vi "Pickering_action.vi"(0 "Pickering status":path=path "C:/LabView/PPMS basic VIs/Switch Status.txt", 1 "Array":T2(array[cluster])=[{"Channel x"="x12", "Channel y"="y1"}, {"Channel x"="x12", "Channel y"="y2"}, {"Channel x"="x12", "Channel y"="y3"}, {"Channel x"="x12", "Channel y"="y4"}, {"Channel x"="x12", "Channel y"="y5"}, {"Channel x"="x12", "Channel y"="y6"}, {"Channel x"="x12", "Channel y"="y7"}, {"Channel x"="x12", "Channel y"="y8"}], 2 "option string":string="Simulate=0,RangeCheck=1,QueryInstrStatus=0,Cache=1,DriverSetup=Model:40-726-511-M;", 3 "Action":u16(ring) items=["Close", "Open", "Disconnect all"], 4 "Initialize":bool, 5 "resource name":string="PXI9::13::INSTR") -> (7 "instrument handle out":refnum<k15>="PXI9::13::INSTR (2)")   [LabVIEW 2011]
panel:
  out "Additionally Connected Switches":T1(array[cluster])=[{"result string"="xA5", "result string"="yA7"}, {"result string"="comC5", "result string"="chC5"}, {"result string"="comD7", "result string"="chD7"}, {"result string"="xA8", "result string"="yA4"}, {"result string"="xA8", "result string"="yA8"}, {"result string"="comC8", "result string"="chC8"}, {"result string"="xA1", "result string"="yA3"}, {"result string"="comD3", "result string"="chD3"}, {"result string"="xA3", "result string"="yA5"}, {"result string"="comC3", "result string"="chC3"}, {"result string"="comD5", "result string"="chD5"}]
  out "Disconnected Switches":T1(array[cluster])=[{"result string"="xA12", "result string"="yA1"}, {"result string"="comB12", "result string"="chB12"}, {"result string"="xA12", "result string"="yA2"}, {"result string"="comE2", "result string"="chE2"}, {"result string"="xA12", "result string"="yA3"}, {"result string"="comE3", "result string"="chE3"}, {"result string"="xA12", "result string"="yA4"}, {"result string"="xA12", "result string"="yA5"}, {"result string"="comC12", "result string"="chC12"}, {"result string"="comE5", "result string"="chE5"}, {"result string"="xA12", "result string"="yA6"}, {"result string"="comE6", "result string"="chE6"}, {"result string"="xA12", "result string"="yA7"}, {"result string"="comE7", "result string"="chE7"}, {"result string"="xA12", "result string"="yA8"}, {"result string"="xA1", "result string"="yA1"}, {"result string"="comD1", "result string"="chD1"}, {"result string"="xA2", "result string"="yA1"}, {"result string"="comB2", "result string"="chB2"}, {"result string"="xA3", "result string"="yA1"}, {"result string"="comB3", "result string"="chB3"}, {"result string"="xA4", "result string"="yA1"}, {"result string"="comB4", "result string"="chB4"}, {"result string"="xA5", "result string"="yA1"}, {"result string"="comB5", "result string"="chB5"}, {"result string"="xA6", "result string"="yA1"}, {"result string"="comB6", "result string"="chB6"}, {"result string"="xA8", "result string"="yA1"}, {"result string"="xA9", "result string"="yA1"}, {"result string"="comB9", "result string"="chB9"}, {"result string"="xA10", "result string"="yA1"}, {"result string"="comB10", "result string"="chB10"}, {"result string"="xA11", "result string"="yA1"}, {"result string"="comB11", "result string"="chB11"}]
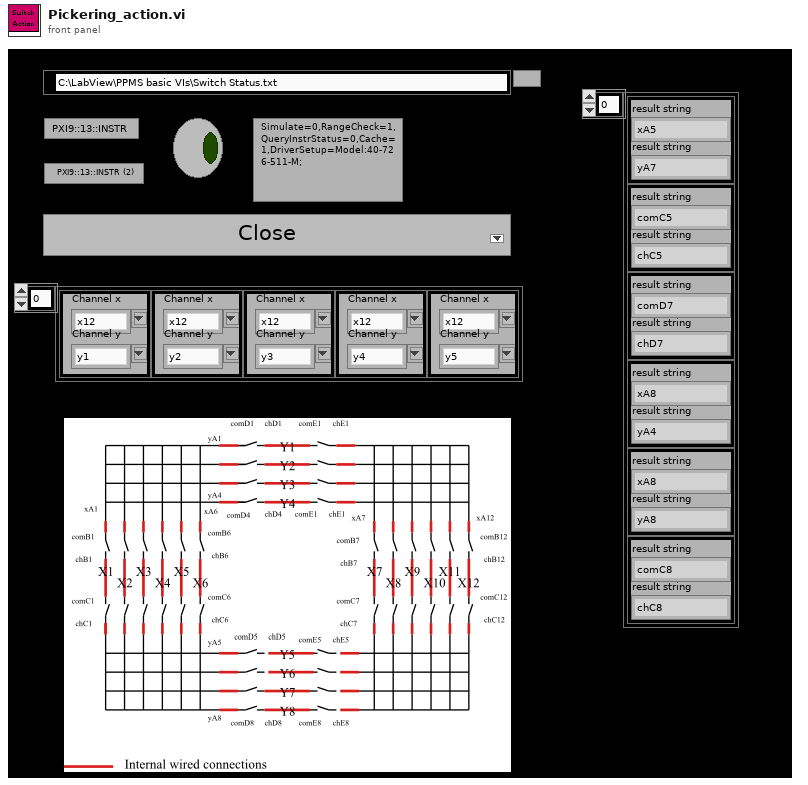
[diagram p1: front panel]
types:
  T1 = cluster{"result string":string, "result string":string}[]
  T2 = cluster{"Channel x":string, "Channel y":string}[]
  T3 = cluster{"output string":string, "output string":string}
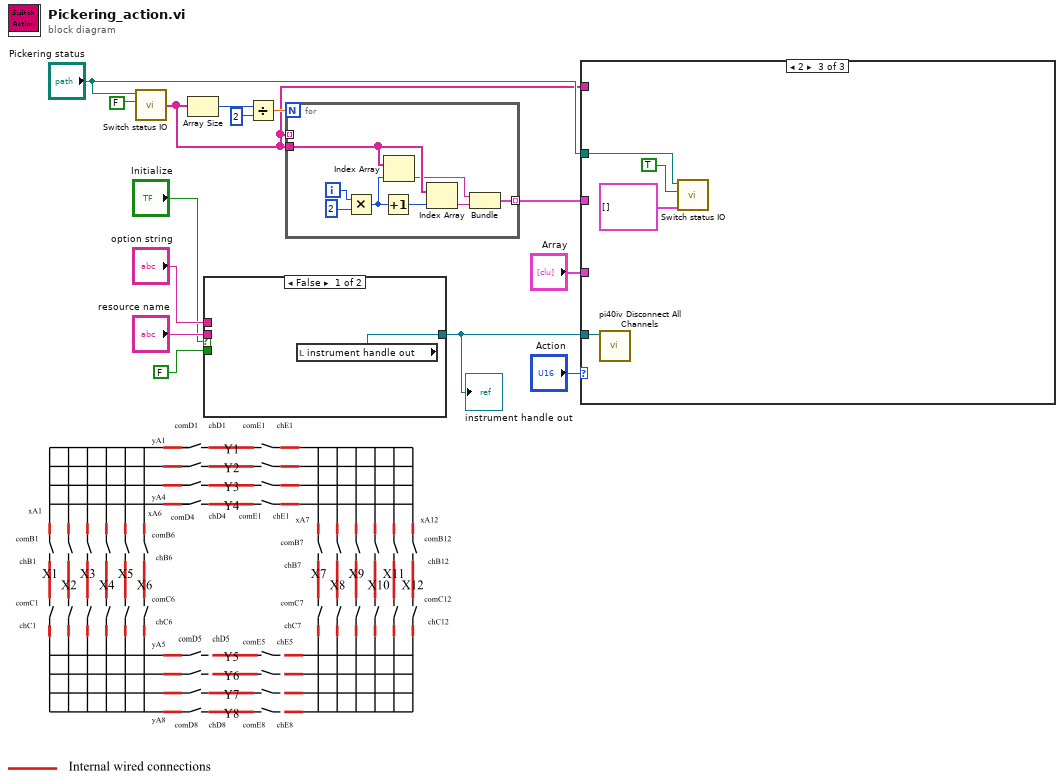
[diagram p0: block diagram]
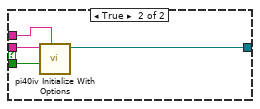
[diagram p2: hidden frame]
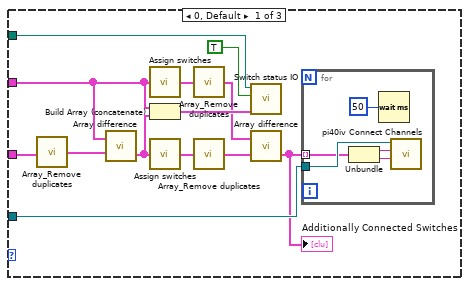
[diagram p3: hidden frame]
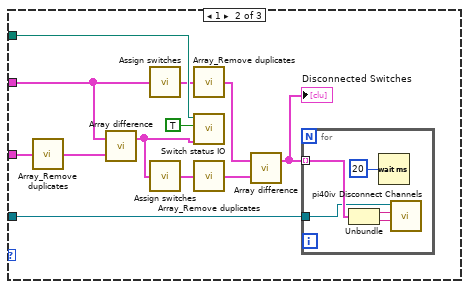
[diagram p4: hidden frame]
diagram:
  n1 = call "Switch status IO.vi"("Write: T\nRead: F"=FALSE ("Write: T\nRead: F"), "Path"="Pickering status") -> ("String out"=w3:string[])  [unwired: 4 in]
  n2 = Array Size(array=w3) -> (size(s)=w8:i32)
  n3 = case shown="False" "Initialize" {
    tunnel: "resource name" -> [_ w19]
    tunnel: "option string" -> [_ w18]
    tunnel: FALSE ("reset device") -> [_ w17]
    tunnel: [w15 w16] -> w1
    frame False {
      n4 = local read "instrument handle out"() -> (w15:refnum<k15>)
    }
    frame True {
      n5 = call <instrlib>:"pi40iv Initialize With Options.vi"("option string"=w18, "reset device"=w17, "resource name"=w19) -> ("instrument handle out"=w16:refnum<k15>)  [unwired: 7 in, 1 out]
    }
  }
  "instrument handle out" <- w1
  n6 = Divide(x=w8, y=2) -> (x/y=w6:dbl)
  n7 = for {
    N: w6 -> [_]
    tunnel: w3 -> [w27]
    tunnel: w3 -> [_] mode=indexing
    tunnel: [w23] -> w5 mode=indexing
    i -> [w22]
    n8 = Multiply(x=w22, y=2) -> (x*y=w20:i32)
    n9 = Increment(x=w20) -> (x+1=w26:i32)
    n10 = Index Array(array=w27, index=w20) -> (element=w25:string)
    n11 = Index Array(array=w27, index=w26) -> (element=w24:string)
    n12 = Bundle("output string"=w25, "output string"=w24) -> (w23:T3)  [unwired: 1 in]
  }
  n13 = case shown="2" "Action" {
    tunnel: w1 -> [w40 w52 w66]
    tunnel: "Array" -> [w29 w47 _]
    tunnel: w3 -> [_ _ _]
    tunnel: "Pickering status" -> [w39 w56 w65]
    tunnel: w5 -> [w34 w51 _]
    frame 0, Default {
      n14 = call "Array_Remove duplicates.vi"("Array Input"=w29) -> ("Array Output"=w28:T1)
      n15 = call "Array difference.vi"("Array 2"=w28, "Array 1"=w34) -> ("Array 2-(array1&2)"=w36:cluster{"String":string, "String 2":string}[])  [unwired: 1 out]
      n16 = call "Assign switches.vi"("Array"=w34) -> ("Array 2"=w33:T1)
      n17 = Build Array (concatenate)(w34, w36) -> (w37:cluster{"String":string, "String 2":string}[])
      n18 = call "Assign switches.vi"("Array"=w36) -> ("Array 2"=w35:T1)
      n19 = call "Array_Remove duplicates.vi"("Array Input"=w33) -> ("Array Output"=w32:T1)
      n20 = call "Array_Remove duplicates.vi"("Array Input"=w35) -> ("Array Output"=w31:T1)
      n21 = call "Switch status IO.vi"("String input"=w37, "Write: T\nRead: F"=TRUE ("Write: T\nRead: F"), "Path"=w39) -> ()  [unwired: 3 in, 1 out]
      n22 = call "Array difference.vi"("Array 2"=w31, "Array 1"=w32) -> ("Array 2-(array1&2)"=w30:cluster{"String":string, "String 2":string}[])  [unwired: 1 out]
      "Additionally Connected Switches" <- w30
      n23 = for {
        tunnel: w40 -> [w45]
        tunnel: w30 -> [w44] mode=indexing
        n24 = Unbundle(w44) -> ("String"=w43:string, "String 2"=w42:string)
        n25 = Wait (ms)(milliseconds to wait=u32 50) -> ()  [unwired: 1 out]
        n26 = call <instrlib>:"pi40iv Connect Channels.vi"("channel 2"=w42, "channel 1"=w43, "instrument handle"=w45) -> ()  [unwired: 7 in, 2 out]
      }
    }
    frame 1 {
      n27 = call "Array_Remove duplicates.vi"("Array Input"=w47) -> ("Array Output"=w46:T1)
      n28 = call "Array difference.vi"("Array 2"=w46, "Array 1"=w51) -> ("Array 1-(array1&2)"=w49:cluster{"String":string, "String 2":string}[])  [unwired: 1 out]
      n29 = call "Assign switches.vi"("Array"=w51) -> ("Array 2"=w50:T1)
      n30 = call "Assign switches.vi"("Array"=w49) -> ("Array 2"=w48:T1)
      n31 = call "Array_Remove duplicates.vi"("Array Input"=w50) -> ("Array Output"=w55:T1)
      n32 = call "Switch status IO.vi"("String input"=w49, "Write: T\nRead: F"=TRUE ("Write: T\nRead: F"), "Path"=w56) -> ()  [unwired: 3 in, 1 out]
      n33 = call "Array_Remove duplicates.vi"("Array Input"=w48) -> ("Array Output"=w54:T1)
      n34 = call "Array difference.vi"("Array 2"=w54, "Array 1"=w55) -> ("Array 1-(array1&2)"=w53:cluster{"String":string, "String 2":string}[])  [unwired: 1 out]
      "Disconnected Switches" <- w53
      n35 = for {
        tunnel: w53 -> [w62] mode=indexing
        tunnel: w52 -> [w59]
        n36 = Unbundle(w62) -> ("String"=w61:string, "String 2"=w60:string)
        n37 = Wait (ms)(milliseconds to wait=u32 20) -> ()  [unwired: 1 out]
        n38 = call <instrlib>:"pi40iv Disconnect Channels.vi"("channel 2"=w60, "channel 1"=w61, "instrument handle"=w59) -> ()  [unwired: 7 in, 2 out]
      }
    }
    frame 2 {
      n39 = call <instrlib>:"pi40iv Disconnect All Channels.vi"("instrument handle"=w66) -> ()  [unwired: 9 in, 2 out]
      n40 = call "Switch status IO.vi"("String input"=T1 [], "Write: T\nRead: F"=TRUE ("Write: T\nRead: F"), "Path"=w65) -> ()  [unwired: 3 in, 1 out]
    }
  }
